vi "HoloTrackerLauncher.vi"   [LabVIEW 2023]
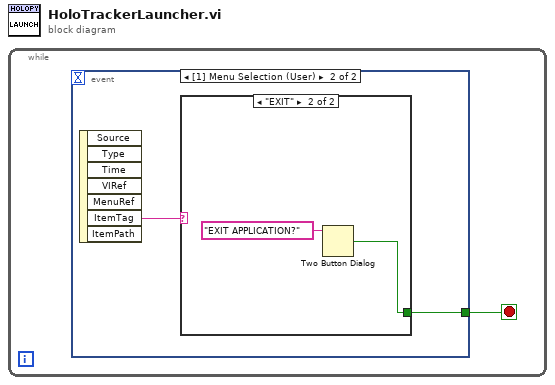
[diagram p0: block diagram]
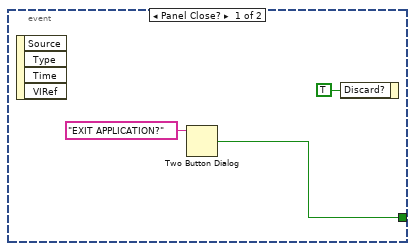
[diagram p2: hidden frame]
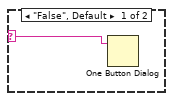
[diagram p3: hidden frame]
diagram:
  n1 = while {
    stop <- w1 stop-if-true
    n2 = event shown="[1] Menu Selection (User)" {
      selector: _ -> [_ _]
      dyn-events: _ -> [_ _]
      timeout: _ -> [_ _]
      tunnel: [w3 w5] -> w1
      event Panel Close? {
        n3 = event-data() -> ()  [unwired: 1 in, 4 out]
        n4 = Two Button Dialog(message="EXIT APPLICATION?") -> (T button?=w3:bool)  [unwired: 2 in]
        n5 = event-data("Discard?"=TRUE) -> ()  [unwired: 1 in, 1 out]
      }
      event Menu Selection (User) {
        n6 = event-data() -> ("ItemTag"=w6:string)  [unwired: 1 in, 6 out]
        n7 = case shown="\"EXIT\"" w6 {
          selector: w6 -> [w7 _]
          tunnel: [_ w8] -> w5
          frame "False", Default {
            n8 = One Button Dialog(message=w7) -> ()  [unwired: 1 in, 1 out]
          }
          frame "EXIT" {
            n9 = Two Button Dialog(message="EXIT APPLICATION?") -> (T button?=w8:bool)  [unwired: 2 in]
          }
        }
      }
    }
  }
